vi "writeDelay.vi"(8 "error in (no error)":errorcluster, 10 "Delay(us)":u32, 11 "ModbusBuffer in":refnum<class "ModbusBufferBuilder.lvclass">) -> (0 "error out":errorcluster, 3 "ModbusBuffer out":refnum<class "ModbusBufferBuilder.lvclass">)   [LabVIEW 2016, in "ModbusBufferBuilder.lvclass"]
uses:
  ModbusBufferBuilder.lvclass
  ModbusBufferBuilder.lvclass/ModbusBufferBuilder.ctl
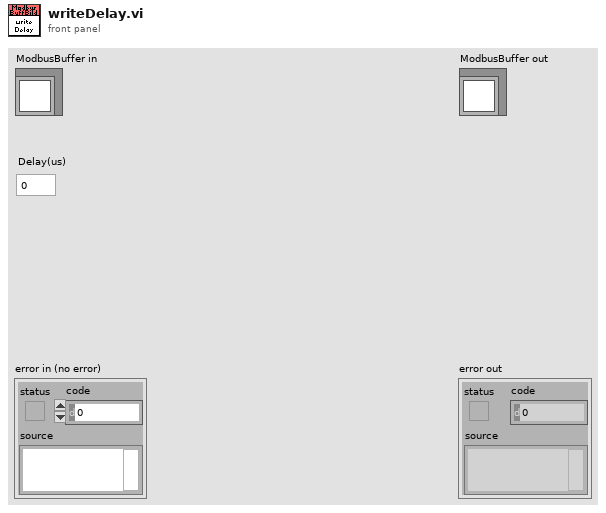
[diagram p1: front panel]
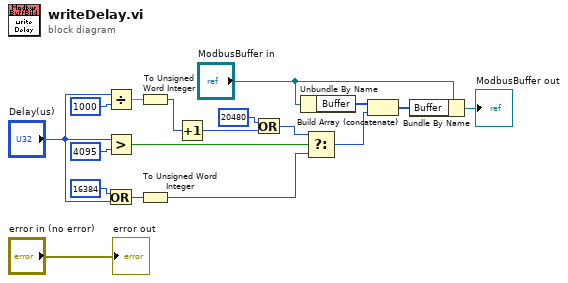
[diagram p0: block diagram]
diagram:
  n1 = Divide(x="Delay(us)", y=u32 1000) -> (x/y=w16:dbl)
  n2 = Greater?(x="Delay(us)", y=u32 4095) -> (0:w14:bool)
  n3 = Or(x=u16 16384, y="Delay(us)") -> (x .or. y?=w7:u32)
  n4 = To Unsigned Word Integer(number=w16) -> (unsigned 16bit integer=w13:u16)
  n5 = To Unsigned Word Integer(number=w7) -> (unsigned 16bit integer=w15:u16)
  n6 = Increment(x=w13) -> (x+1=w6:u16)
  n7 = Or(x=u16 20480, y=w6) -> (x .or. y?=w4:u16)
  n8 = Unbundle By Name("ModbusBuffer in") -> ("Buffer"=w3:u16[])
  n9 = Select(t=w4, s=w14, f=w15) -> (s? t:f=w2:u16)
  n10 = Build Array (concatenate)(w3, w2) -> (w1:u16[])
  n11 = Bundle By Name(cluster="ModbusBuffer in", "Buffer"=w1) -> (→"ModbusBuffer out":refnum<class "ModbusBufferBuilder.lvclass">)
  "error out" <- "error in (no error)"
